vi "TestReadWrite_DEPRECATED.vi"() -> ()   [LabVIEW 2017]
uses:
  Definitions/Dictionary--Cluster.ctl
  Definitions/Private/Font -- Cluster.ctl
  Definitions/Private/Phrase Dictionary Entry -- Cluster.ctl
  API/JKI Simple Localization.lvlib
panel:
  out "ASCII String":string
  out "JSON String":string
  out "x = y?":bool
  out "Dictionary":T1
  out "error out":errorcluster
  in  "Dictionary File Path":path
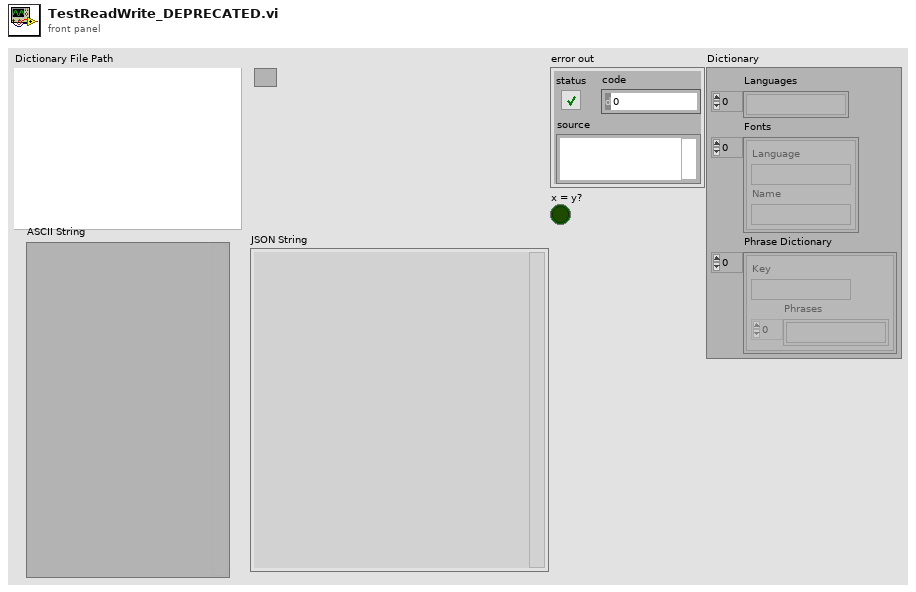
[diagram p1: front panel]
types:
  T1 = typedef "JKI Simple Localization.lvlib/Dictionary--Cluster.ctl" = cluster{"Languages":string[], "Fonts":T2[], "Phrase Dictionary":T3[]}
  T2 = typedef "JKI Simple Localization.lvlib/Font -- Cluster.ctl" = cluster{"Language":string, "Name":string}
  T3 = typedef "JKI Simple Localization.lvlib/Phrase Dictionary Entry -- Cluster.ctl" = cluster{"Key":string, "Phrases":string[]}
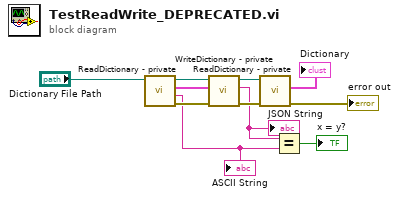
[diagram p0: block diagram]
diagram:
  n1 = call "ReadDictionary - private.vi"("Dictionary File Path"="Dictionary File Path") -> ("error out"=w9:errorcluster, "ASCII String"=w1:string, "Dictionary"=w10:T1, "Dictionary File Path out"=w11:path)  [unwired: 7 in]
  "ASCII String" <- w1
  n2 = call "WriteDictionary - private.vi"("error in (no error)"=w9, "Localization"=w10, "Dictionary Path"=w11) -> ("error out"=w6:errorcluster, "JSON String"=w3:string, "Dictionary Path Dup"=w7:path)  [unwired: 6 in]
  "JSON String" <- w3
  n3 = call "ReadDictionary - private.vi"("error in (no error)"=w6, "Dictionary File Path"=w7) -> ("error out"=→"error out":errorcluster, "Dictionary"=→"Dictionary":T1)  [unwired: 6 in, 2 out]
  n4 = Equal?(x=w3, y=w1) -> (x = y?=→"x = y?":bool)
